vi "SetSP.vi"(8 "error in (no error)":errorcluster, 10 "ctlSP":dbl[](array[numeric]), 11 "CN79000 in":refnum<class "CN79000.lvclass">=refnum) -> (0 "error out":errorcluster, 3 "CN79000 out":refnum<class "CN79000.lvclass">)   [LabVIEW 2014, in "CN79000.lvclass"]
uses:
  CN79000.lvclass
  Build Command-Multi Val.vi
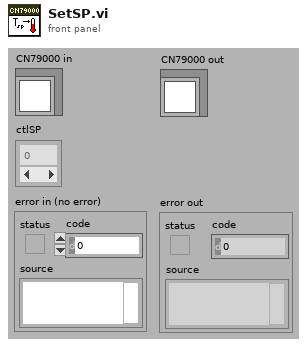
[diagram p1: front panel]
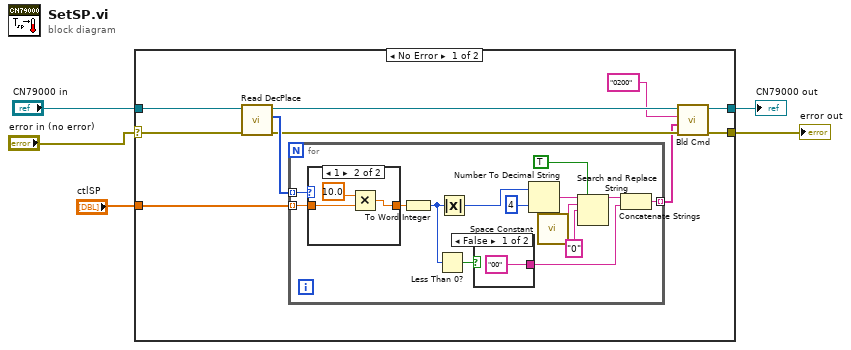
[diagram p0: block diagram]
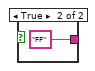
[diagram p3: hidden frame]
diagram:
  n1 = case shown="No Error" "error in (no error)" {
    selector: "error in (no error)" -> [w12 w37]
    tunnel: [w6 w37] -> w5
    tunnel: [w7 w36] -> w3
    tunnel: "CN79000 in" -> [w15 w36]
    tunnel: "ctlSP" -> [w13 _]
    frame No Error {
      n2 = call "Read DecPlace.vi"("error in"=w12, "CN79000 in"=w15) -> ("error out"=w10:errorcluster, "DecPt"=w14:i32[], "CN79000 out"=w11:refnum<class "CN79000.lvclass">)  [unwired: 7 in]
      n3 = for {
        tunnel: w14 -> [w17] mode=indexing
        tunnel: w13 -> [w18] mode=indexing
        tunnel: [w16] -> w9 mode=indexing
        n4 = case shown="1" w17 {
          tunnel: w18 -> [w30 w33]
          tunnel: [w30 w31] -> w20
          frame 0, Default {
          }
          frame 1 {
            n5 = Multiply(x=10.0, y=w33) -> (x*y=w31:dbl)
          }
        }
        n6 = To Word Integer(number=w20) -> (16bit integer=w19:i16)
        n7 = Less Than 0?(x=w19) -> (x < 0?=w27:bool)
        n8 = Absolute Value(x=w19) -> (abs(x)=w21:i16)
        n9 = case shown="False" w27 {
          tunnel: ["00" "FF"] -> w29
          frame False {
          }
          frame True {
          }
        }
        n10 = Number To Decimal String(number=w21, width (-)=i16 4) -> (decimal integer string=w23:string)
        n11 = call <vilib>:"Space Constant.vi"() -> ("String"=w24:string)
        n12 = Search and Replace String(replace all?=TRUE ("replace all? (F)"), input string=w23, search string=w24, replace string="0" ("search string")) -> (result string=w28:string)  [unwired: 4 in, 3 out]
        n13 = Concatenate Strings(w28, w29) -> (w16:string)
      }
      n14 = call-poly "Bld Cmd.vi"("error in"=w10, "Val"=w9, "Cmd"="0200", "CN79000 in"=w11) -> ("error out"=w6:errorcluster, "CN79000 out"=w7:refnum<class "CN79000.lvclass">)  [unwired: 3 in, 2 out]
    }
    frame Error {
    }
  }
  "error out" <- w5
  "CN79000 out" <- w3
